vi "Search from PRN  & Replacement Data.vi"(9 "Serial N0":i32, 11 "Prn File Call":string) -> (1 "Final Serial No":string, 2 "Line Name":i32, 3 "Send on Barcode TSC-TA310":string)   [LabVIEW 2015]
panel:
  out "concatenated string":string
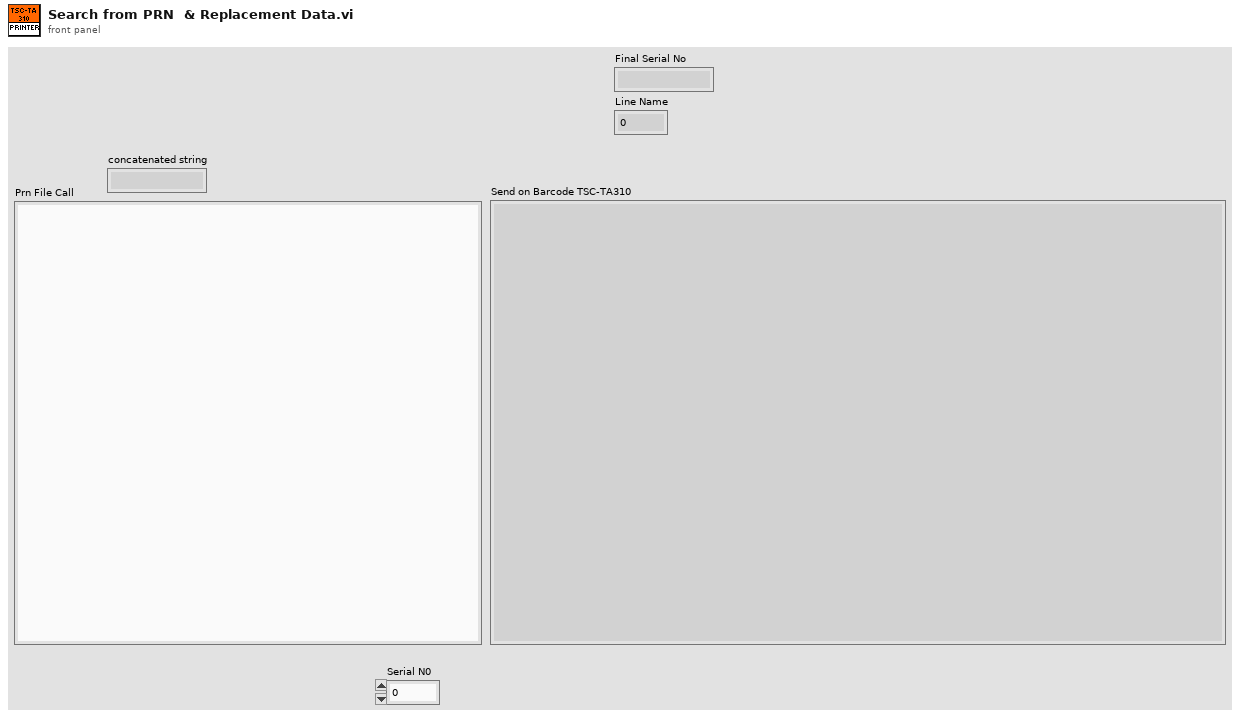
[diagram p1: front panel]
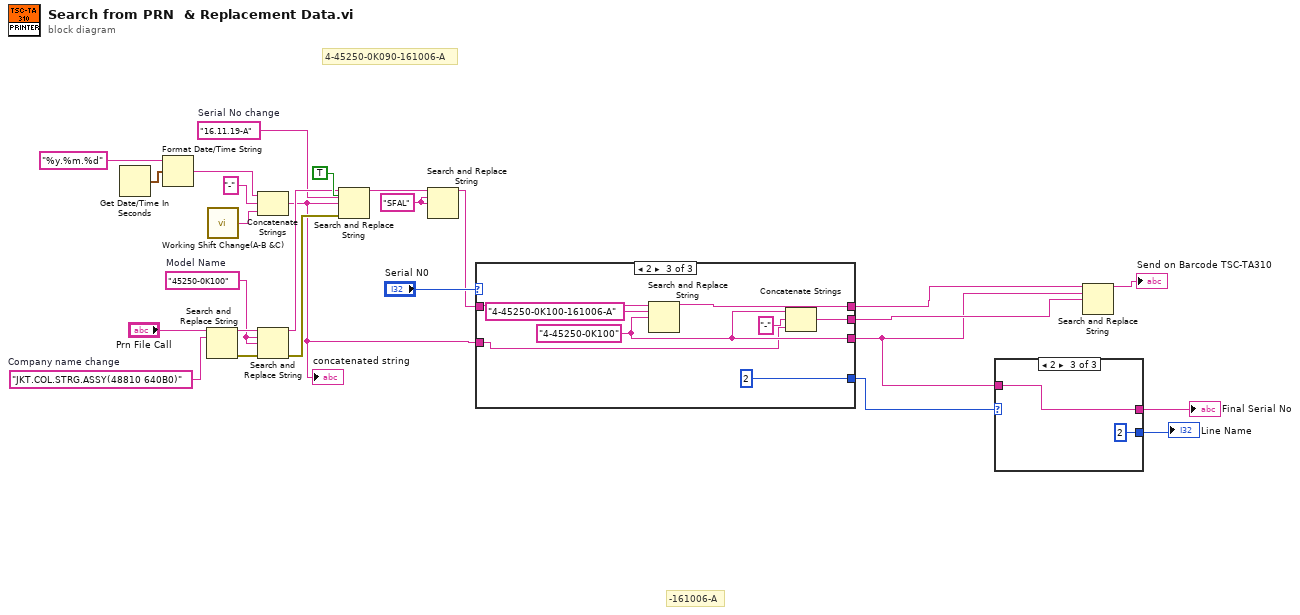
[diagram p0: block diagram]
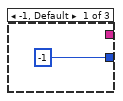
[diagram p2: hidden frame]
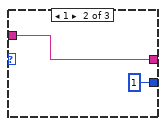
[diagram p3: hidden frame]
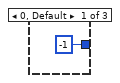
[diagram p4: hidden frame]
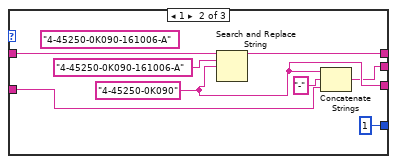
[diagram p5: hidden frame]
diagram:
  w17 = "SFAL" ("search string")
  w14 = "45250-0K100"  # Model Name
  w18 = "16.11.19-A"  # Serial No change
  w23 = "JKT.COL.STRG.ASSY(48810 640B0)"  # Company name change
  # "4-45250-0K090-161006-A"
  # "-161006-A"
  n1 = Get Date/Time In Seconds() -> (seconds since 1Jan1904=w25:timestamp)
  n2 = Format Date/Time String(time format string (%c)="%y.%m.%d", seconds (now)=w25) -> (date/time string=w13:string)  [unwired: 1 in]
  n3 = Search and Replace String(input string="Prn File Call", search string=w23) -> (result string=w22:string, error out=w21:errorcluster)  [unwired: 6 in, 2 out]
  n4 = call "Working Shift Change(A-B &C).vi"() -> ("Shift Change"=w15:string)  [unwired: 9 in]
  n5 = Concatenate Strings(w13, "-" ("string"), w15) -> (w6:string)
  "concatenated string" <- w6
  n6 = Search and Replace String(input string=w22, search string=w14, replace string=w14, error in=w21) -> (result string=w20:string, error out=w19:errorcluster)  [unwired: 4 in, 2 out]
  n7 = Search and Replace String(replace all?=TRUE ("replace all? (F)"), input string=w20, search string=w18, replace string=w6, error in=w19) -> (result string=w12:string)  [unwired: 3 in, 3 out]
  n8 = Search and Replace String(input string=w12, search string=w17, replace string=w17) -> (result string=w8:string)  [unwired: 5 in, 3 out]
  n9 = case shown="2" "Serial N0" {
    tunnel: [_ w33 w42] -> w7
    tunnel: w8 -> [_ w34 w41]
    tunnel: [_ w30 w39] -> w3
    tunnel: w6 -> [_ w31 w38]
    tunnel: [_ w29 w37] -> w5
    tunnel: [-1 1 2] -> w2
    frame 0, Default {
    }
    frame 1 {
      w30 = "4-45250-0K090" ("search string")
      (unwired) "4-45250-0K090-161006-A" ("search string")
      n10 = Search and Replace String(input string=w34, search string="4-45250-0K090-161006-A", replace string=w30) -> (result string=w33:string)  [unwired: 5 in, 3 out]
      n11 = Concatenate Strings(w30, "-" ("string"), w31) -> (w29:string)
    }
    frame 2 {
      w39 = "4-45250-0K100" ("search string")
      n12 = Search and Replace String(input string=w41, search string="4-45250-0K100-161006-A", replace string=w39) -> (result string=w42:string)  [unwired: 5 in, 3 out]
      n13 = Concatenate Strings(w39, "-" ("string"), w38) -> (w37:string)
    }
  }
  n14 = case shown="2" w2 {
    tunnel: [_ w46 w48] -> w4
    tunnel: w3 -> [_ w46 w48]
    tunnel: [-1 1 2] -> w1
    frame -1, Default {
    }
    frame 1 {
    }
    frame 2 {
    }
  }
  "Final Serial No" <- w4
  "Line Name" <- w1
  n15 = Search and Replace String(input string=w7, search string=w3, replace string=w5) -> (result string=→"Send on Barcode TSC-TA310":string)  [unwired: 5 in, 3 out]
